vi "VSI Write Read Bytes.vi"(0 "DevType":i32, 1 "WriteLen":u16, 5 "DevIndex":i32, 7 "SPIIndex":i32, 9 "pWriteData":string, 11 "error in (no error)":errorcluster, 12 "ReadLen":u16) -> (4 "pReadData":string, 6 "function return":i32, 10 "pWriteData out":string, 15 "error out":errorcluster)   [LabVIEW 2012, in "ControlSPI.lvlib"]
doc: "int WINAPI VSI_WriteReadBytes(int DevType,int DevIndex,int SPIIndex,unsigned char* pWriteData,unsigned short WriteLen,unsigned char * pReadData,unsigned short ReadLen);"
uses:
  ControlSPI.lvlib
  Ginkgo_Driver.dll
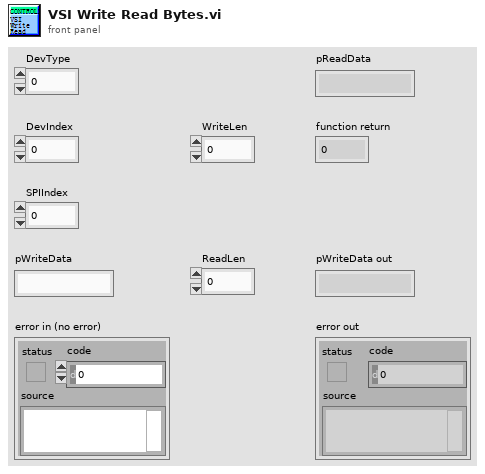
[diagram p1: front panel]
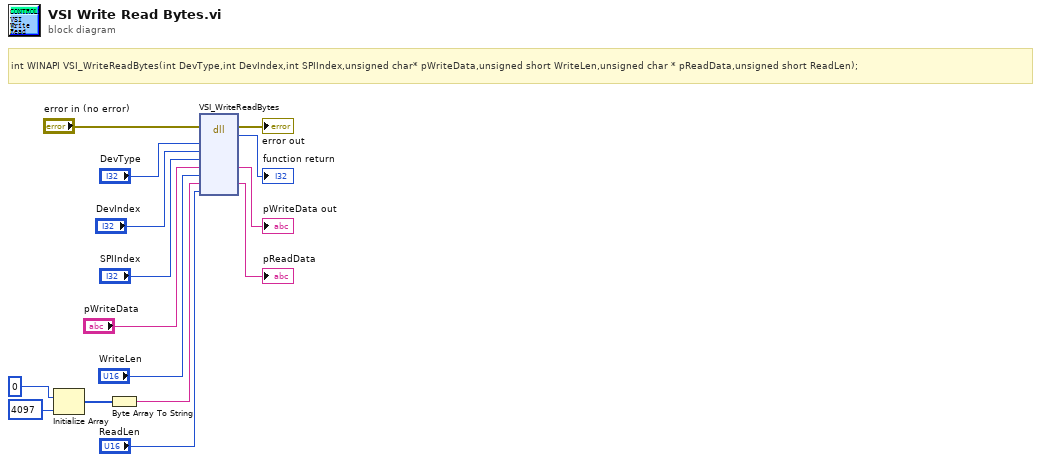
[diagram p0: block diagram]
diagram:
  # "int WINAPI VSI_WriteReadBytes(int DevType,int DevIndex,int SPIIndex,unsigned char* pWriteData,unsigned short WriteLen,unsigned char * pReadData,unsigned short ReadLen);"
  n1 = Initialize Array(u8 0 ("element"), 4097 ("dimension size")) -> (w8:u8[])
  n2 = Byte Array To String(unsigned byte array=w8) -> (string=w7:string)
  n3 = dll-call lib="E:/Project/vt_ginkgo/truck/Ginkgo Driver/vs2010/Ginkgo_USB-I2C_API_v2.0.3.0/lib/labview_64bit/ControlSPI/Ginkgo_Driver.*" fn="VSI_WriteReadBytes"(error in="error in (no error)", "DevType"="DevType", "DevIndex"="DevIndex", "SPIIndex"="SPIIndex", "pWriteData"="pWriteData", "WriteLen"="WriteLen", "pReadData"=w7, "ReadLen"="ReadLen") -> (error out=→"error out":errorcluster, →"function return":i32, "pWriteData"=→"pWriteData out":string, "pReadData"=→"pReadData":string)  [unwired: 7 in, 1 out]
